vi "Write Update.vi"(8 "error in (no error)":errorcluster, 10 "New Value":variant, 11 "Sync Tag In":refnum<class "Synchronised Tag.lvclass">) -> (0 "error out":errorcluster, 3 "Sync Tag Out":refnum<class "Synchronised Tag.lvclass">)   [LabVIEW 2016, in "Synchronised Tag.lvclass"]
doc: "Checks if the value for the shared variable has changed and updates the variable if it has."
uses:
  Synchronised Tag.lvclass
  Synchronised Tag.lvclass/Synchronised Tag.ctl
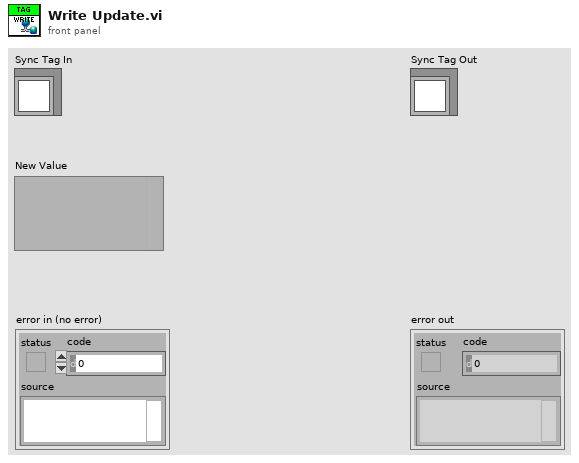
[diagram p1: front panel]
types:
  T1 = typedef "Synchronised Tag.lvclass/Access Mode.ctl" = enum16{"Unused", "Read Only", "Write Only", "Read/Write"}
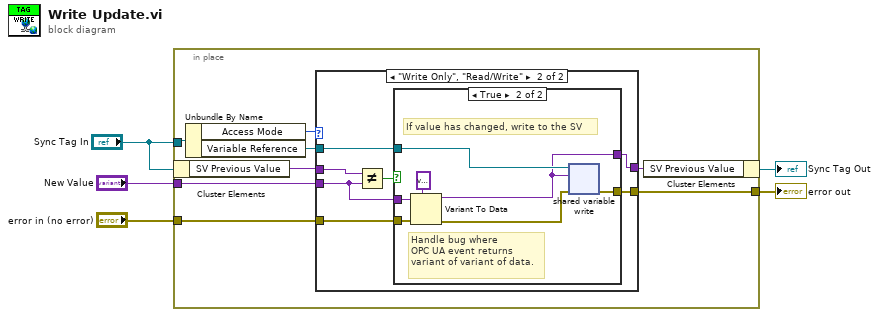
[diagram p0: block diagram]
diagram:
  n1 = in-place {
    in-place-border: "New Value" -> [w13]
    in-place-border: "error in (no error)" -> [w12]
    in-place-border: "Sync Tag In" -> [w9]
    in-place-border: [w6] -> w1
    n2 = in-place-cluster #1("Sync Tag In") -> ("SV Previous Value"=w8:variant)
    n3 = Unbundle By Name(w9) -> ("Access Mode"=w10:T1, "Variable Reference"=w11:refnum<k21>)
    n4 = case shown="\"Write Only\", \"Read/Write\"" w10 {
      tunnel: w8 -> [w14 w22]
      tunnel: w13 -> [_ w20]
      tunnel: w11 -> [_ w19]
      tunnel: w12 -> [w15 w18]
      tunnel: [w15 w17] -> w6
      tunnel: [w14 w16] -> w7
      frame "Unused", "Read Only" {
        # "NOTE: Should we throw a runtime error?"
        # "If writing is unsupported do nothing."
      }
      frame "Write Only", "Read/Write" {
        n5 = Not Equal?(x=w22, y=w20) -> (x != y?=w21:bool)
        n6 = case shown="True" w21 {
          tunnel: w20 -> [w23 w28]
          tunnel: w19 -> [_ w31]
          tunnel: w18 -> [w24 w29]
          tunnel: [w24 w30] -> w17
          tunnel: [w23 w25] -> w16
          frame False {
          }
          frame True {
            # "If value has changed, write to the SV"
            # "Handle bug where\nOPC UA event returns\nvariant of variant of data."
            n7 = Variant To Data(error in=w29, type=variant, Variant=w28) -> (data=w25:variant, error out=w26:errorcluster)
            n8 = shared-variable-write(w31, w26, w25) -> (w30:errorcluster)  [unwired: 1 out]
          }
        }
      }
    }
    n9 = in-place-cluster #1("SV Previous Value"=w7) -> (→"Sync Tag Out":refnum<class "Synchronised Tag.lvclass">)
  }
  "error out" <- w1
